vi "Entry.vi"(8 "error in (no error)":errorcluster, 11 "New State":refnum<class "INIT.lvclass">) -> (0 "error out":errorcluster, 3 "State out":refnum<class "INIT.lvclass">)   [LabVIEW 2021, in "Chef States.lvlib" / "INIT.lvclass"]
doc: "This is an abstract method. Override this method to define the behavior when you enter the state."
uses:
  INIT.lvclass
  Chef State/Chef State.lvclass
  <vilib>/ActorFramework/Actor/Actor.lvclass
  Root Actor Logic/Root Actor Logic Messages/Update State String Msg/Update State String Msg.lvclass
  Chef State Messages/Go to IDLE Msg/Go to IDLE Msg.lvclass
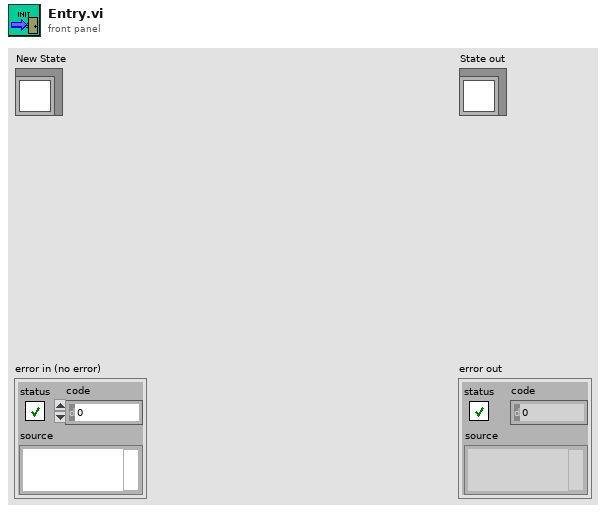
[diagram p1: front panel]
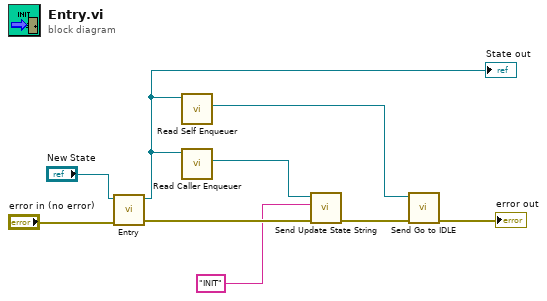
[diagram p0: block diagram]
diagram:
  n1 = call-parent "Entry.vi"("error in (no error)"="error in (no error)", "New State"="New State") -> ("error out"=w9:errorcluster, "State out"=w3:refnum<class "INIT.lvclass">)  [unwired: 8 in]
  "State out" <- w3
  n2 = call <vilib>:"Read Self Enqueuer.vi"("Actor"=w3) -> ("Self Enqueuer"=w1:refnum<class "Message Enqueuer.lvclass">)  [unwired: 10 in]
  n3 = call <vilib>:"Read Caller Enqueuer.vi"("Actor"=w3) -> ("Caller Enqueuer"=w5:refnum<class "Message Enqueuer.lvclass">)  [unwired: 10 in]
  n4 = call "Send Update State String.vi"("error in (no error)"=w9, "State"="INIT", "Message Enqueuer"=w5) -> ("error out"=w6:errorcluster)  [unwired: 7 in, 1 out]
  n5 = call "Send Go to IDLE.vi"("error in (no error)"=w6, "Message Enqueuer"=w1) -> ("error out"=→"error out":errorcluster)  [unwired: 8 in, 1 out]
